vi "Create Initial Stats File.vi"() -> ()   [LabVIEW 2020]
uses:
  WPC Player and Financial Stats.ctl
panel:
  out "error out":errorcluster
  in  "file path (use dialog)":path
  out "appended array":T1[][](array[typedef]) {"Date Updated" format="%<%m/%d/%Y>T"}
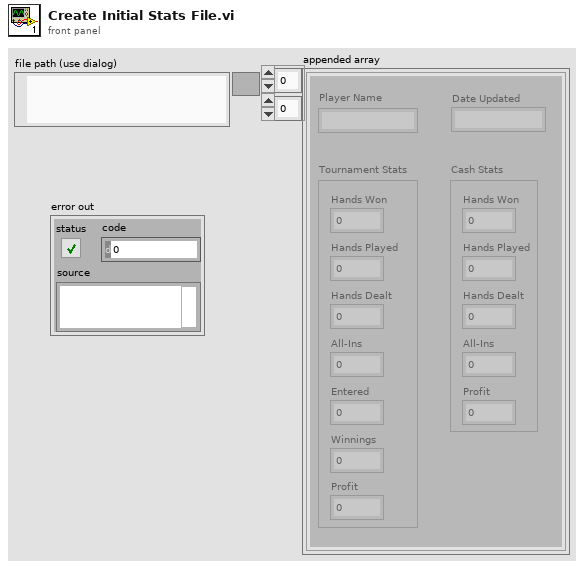
[diagram p1: front panel]
types:
  T1 = typedef "WPC Player and Financial Stats.ctl" = cluster{"Player Name":string, "Date Updated":timestamp, "Tournament Stats":cluster{"Hands Won":u32, "Hands Played":u32, "Hands Dealt":u32, "All-Ins":u32, "Entered":u32, "Winnings":dbl, "Profit":dbl}, "Cash Stats":cluster{"Hands Won":u32, "Hands Played":u32, "Hands Dealt":u32, "All-Ins":u32, "Profit":dbl}}
  T2 = enum16{"open", "replace", "create", "open or create", "replace or create", "replace or create with confirmation"}
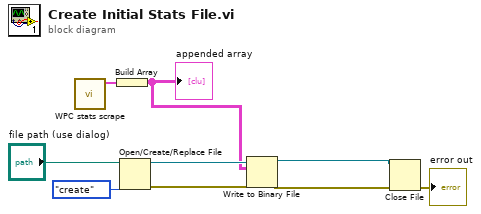
[diagram p0: block diagram]
diagram:
  n1 = call "WPC stats scrape.vi"() -> ("WPC Player Stats"=w9:T1[])  [unwired: 11 in]
  n2 = Build Array(w9) -> (w4:T1[][])
  "appended array" <- w4
  n3 = Open/Create/Replace File(file path (use dialog)="file path (use dialog)", operation (0:open)=T2."create") -> (refnum out=w6:refnum<file>, error out=w5:errorcluster)  [unwired: 4 in, 1 out]
  n4 = Write to Binary File(file (use dialog)=w6, data=w4, error in=w5) -> (refnum out=w3:refnum<file>, error out=w2:errorcluster)  [unwired: 3 in, 1 out]
  n5 = Close File(refnum=w3, error in=w2) -> (error out=→"error out":errorcluster)  [unwired: 1 out]
